vi "EM_CVx_example.vi"() -> ()   [LabVIEW 2013]
uses:
  EM_CVx.lvlib
panel:
  out "posion":sgl
  in  "查询按钮":bool
  in  "选择运行功能":string(combo)="6"
  out "设置位置结果":i32
  in  "绝对位置":dbl=5.0
  in  "停止":bool
  in  "运行按钮":bool
  out "初始化结果":i32
  in  "ID(轴序号)":i32=1
  in  "轴型号":u16(ring) items=["EM-AS90-100C1", "EM-AS90-65C1", "EM-LS90-20CZ", "EM-LS90-20CZ-old", "EM-LSS65-13C1", "EM-LSS65-30C1", "EM-LSS65-50C1", "EM-LSS90-100C1", "EM-LSS90-150C1", "EM-LSS90-200C1", "EM-RP100", "EM-RP40", "EM-RP60"]
  in  "选择串口":u16(ring) items=["COM1", "COM3", "COM6"]
  out "串口句柄":i32
  out "error out":errorcluster
  out "关闭设备结果":i32
  in  "Error In":errorcluster caption="错误输入"
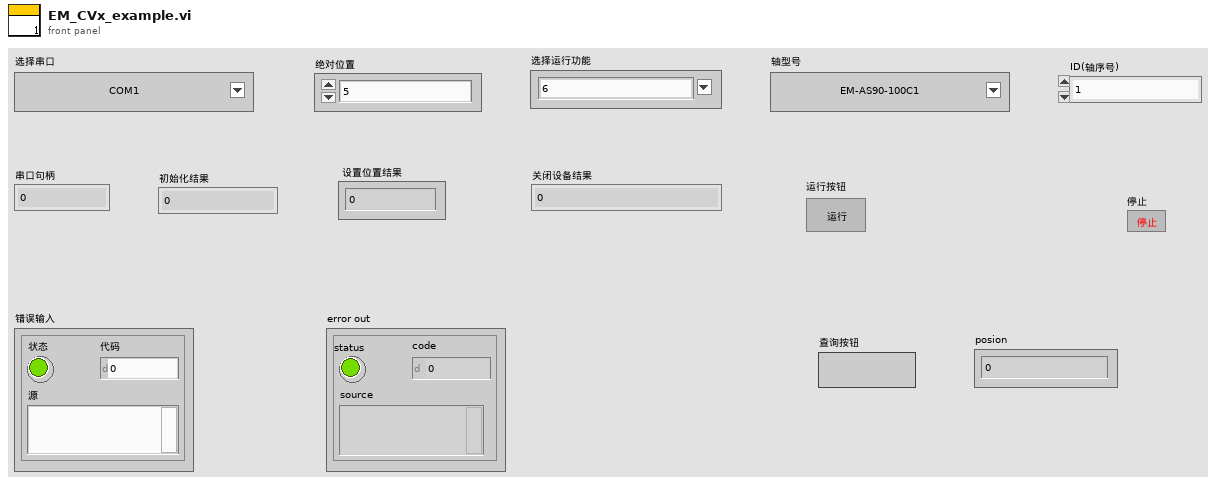
[diagram p1: front panel]
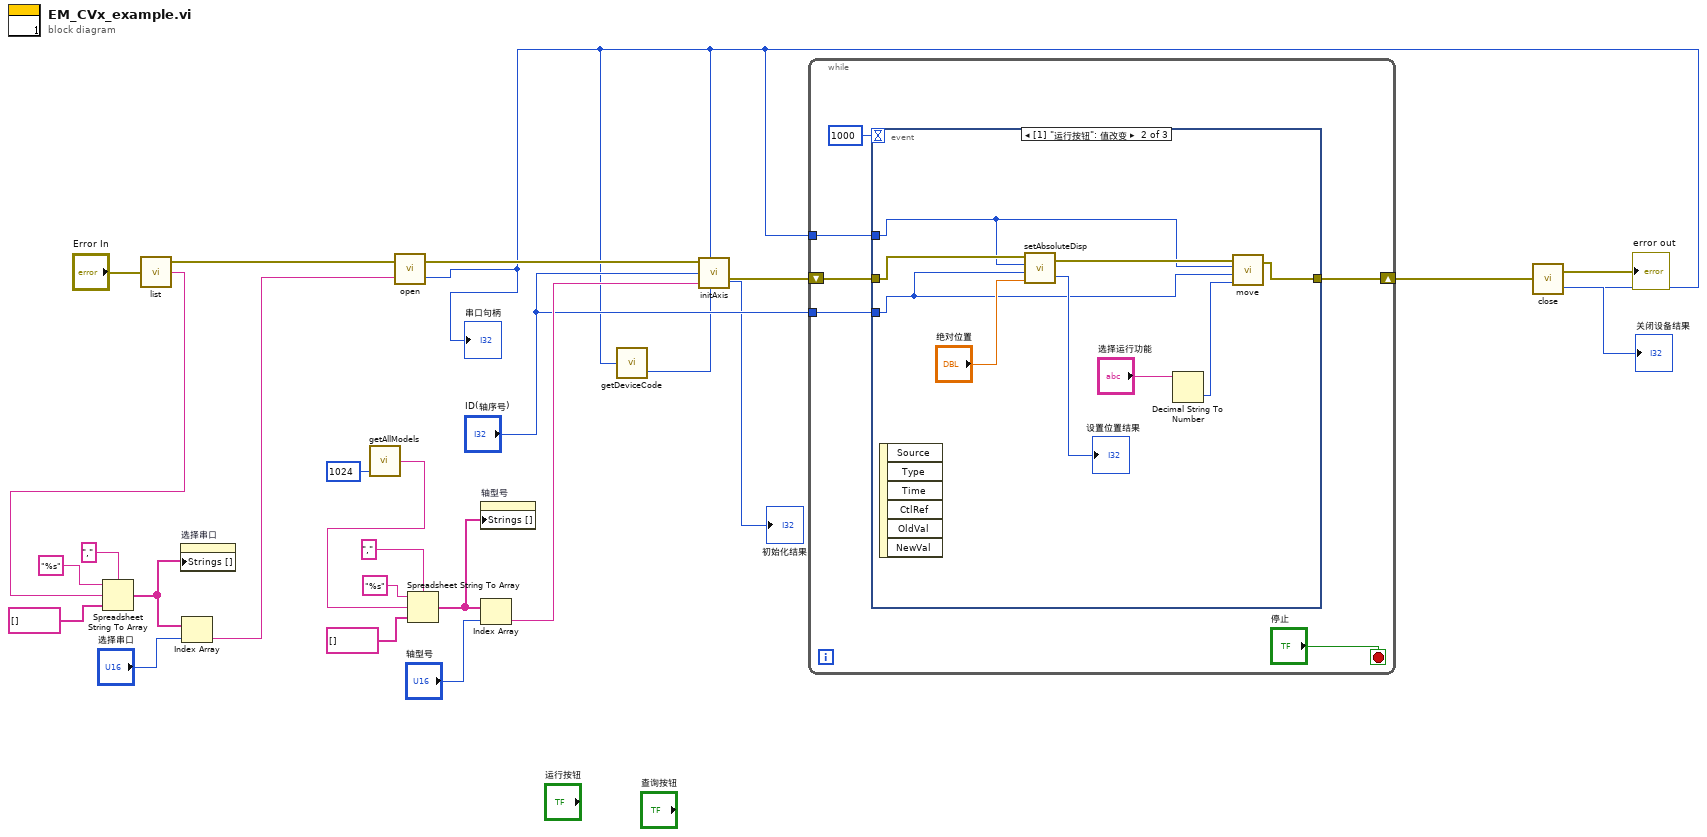
[diagram p0: block diagram]
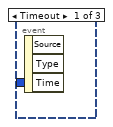
[diagram p2: hidden frame]
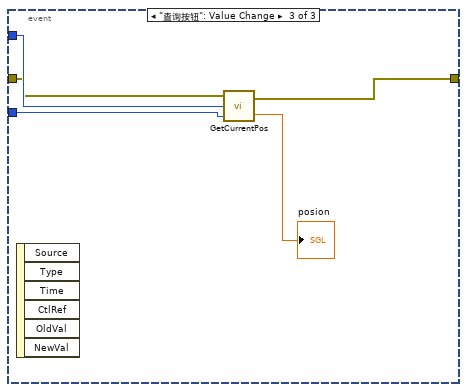
[diagram p3: hidden frame]
diagram:
  n1 = call "list.vi"("error in (no error)"="Error In") -> ("error out"=w24:errorcluster, "serialList"=w17:string)  [unwired: 1 out]
  n2 = Spreadsheet String To Array(delimiter (Tab)="," ("分隔符(Tab)"), format string="%s" ("格式字符串"), spreadsheet string=w17, array type (2D Dbl)=string[] [] ("数组类型(2D Dbl)")) -> (array=w16:string[])
  n3 = property on="选择串口" class="Ring (严格)"("Strings []"=w16) -> ()  [unwired: 2 in, 2 out]
  n4 = Index Array(array=w16, index="选择串口") -> (element=w23:string)
  n5 = call "getAllModels.vi"("len"=1024) -> ("modelNames"=w12:string)  [unwired: 2 in, 2 out]
  n6 = call "open.vi"("serialName"=w23, "Error In"=w24) -> ("返回类型"=w2:i32, "Error Out"=w5:errorcluster)
  "串口句柄" <- w2
  n7 = Spreadsheet String To Array(delimiter (Tab)="," ("分隔符(Tab)"), format string="%s" ("格式字符串"), spreadsheet string=w12, array type (2D Dbl)=string[] [] ("数组类型(2D Dbl)")) -> (array=w9:string[])
  n8 = property on="轴型号" class="Ring (严格)"("Strings []"=w9) -> ()  [unwired: 2 in, 2 out]
  n9 = Index Array(array=w9, index="轴型号") -> (element=w7:string)
  n10 = call "getDeviceCode.vi"("handle"=w2) -> ("return"=w1:i32)  [unwired: 3 in, 1 out]
  n11 = call "initAxis.vi"("Error In"=w5, "handle"=w2, "ID"="ID(轴序号)", "modelName"=w7, "AxisCount"=w1) -> ("Error Out"=w4:errorcluster, "返回类型"=→"初始化结果":i32)
  n12 = while {
    tunnel: "ID(轴序号)" -> [w31]
    tunnel: w2 -> [w29]
    shift-right: [w32] -> w8
    shift-left: w4 -> [w30]
    stop <- "停止" stop-if-true
    n13 = event shown="[1] \"运行按钮\": 值改变" {
      selector: _ -> [_ _ _]
      dyn-events: _ -> [_ _ _]
      timeout: 1000 -> [_ _ _]
      tunnel: [_ w34 w43] -> w32
      tunnel: w31 -> [_ w33 w45]
      tunnel: w30 -> [_ w36 w44]
      tunnel: w29 -> [_ w35 w46]
      event Timeout {
        n14 = event-data() -> ()  [unwired: 1 in, 3 out]
      }
      event "运行按钮": Value Change {
        n15 = event-data() -> ()  [unwired: 1 in, 6 out]
        n16 = call "setAbsoluteDisp.vi"("disp"="绝对位置", "ID"=w33, "handle"=w35, "错误输入（无错误）"=w36) -> ("return"=→"设置位置结果":i32, "错误输出"=w41:errorcluster)
        n17 = Decimal String To Number(string="选择运行功能") -> (number=w38:i32)  [unwired: 2 in, 1 out]
        n18 = call "move.vi"("func"=w38, "ID"=w33, "handle"=w35, "错误输入（无错误）"=w41) -> ("错误输出"=w34:errorcluster)  [unwired: 1 out]
      }
      event "查询按钮": Value Change {
        n19 = event-data() -> ()  [unwired: 1 in, 6 out]
        n20 = call "GetCurrentPos.vi"("ID"=w45, "handle"=w46, "错误输入（无错误）"=w44) -> ("relativeDisp"=→"posion":sgl, "错误输出"=w43:errorcluster)  [unwired: 1 in]
      }
    }
  }
  n21 = call "close.vi"("handle"=w2, "Error In"=w8) -> ("return"=→"关闭设备结果":i32, "Error Out"=→"error out":errorcluster)
